vi "NewProductA.vi"(8 "error in (no error)":errorcluster) -> (0 "error out":errorcluster, 3 "ProductA":refnum<class "ProductA.lvclass">)   [LabVIEW 2020, in "FactoryMethod.lvlib" / "FactoryMethodLazyEvaluation.lvlib" / "ProductA.lvclass"]
uses:
  ProductA.lvclass
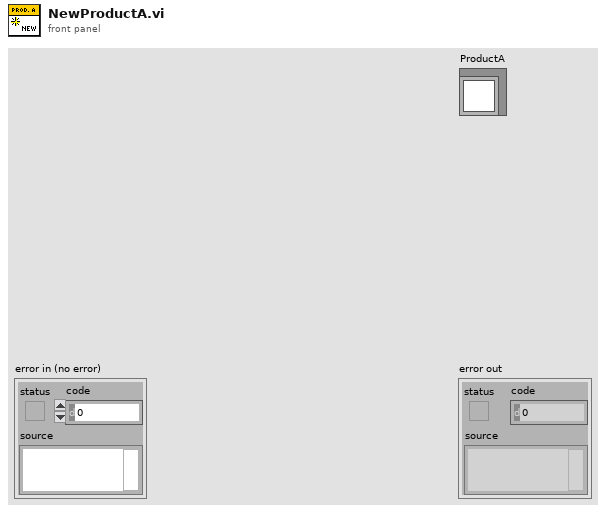
[diagram p1: front panel]
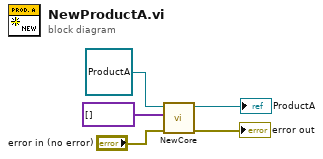
[diagram p0: block diagram]
diagram:
  n1 = call-dynamic "NewCore.vi"("error in (no error)"="error in (no error)", "ParamsArray"=variant[] [], "ProductA"=refnum<class "ProductA.lvclass"> refnum ("ConcreteProductA in")) -> ("error out"=→"error out":errorcluster, "ProductA"=→"ProductA":refnum<class "ProductA.lvclass">)  [unwired: 7 in]
